vi "FIB profile.vi"(4 "Capella HV Data Output":T2 {"Column Vac (Torr)" format="%.2e"; "Gun Vac (Torr)" format="%.2e"; "Lens2 Actual (V)" format="%.1f"; "Lens1 Actual (V)" format="%.1f"; "Emission Actual (uA)" format="%.3f"; "Extrator Actual (V)" format="%.1f"; "Tip Lifetime (uAhr)" format="%.2f"; "Lens2 Target (V)" format="%.1f"; "Lens1 Target (V)" format="%.1f"; "SuppI (uA)" format="%.3f"; "Suppressor (V)" format="%.1f"; "Emission Target (uA)" format="%.3f"; "Extrator Target (V)" format="%.1f"; "Accelerator Actual (V)" format="%.1f"; "Accelerator Target (V)" format="%.1f"; "Filament (A)" format="%.2f"}, 5 "HV Data Output":T3 {"Tip Lifetime (hr)" format="%.2f"; "Lens2I (uA)" format="%.3f"; "Lens2 (V)" format="%.1f"; "Lens1I (uA)" format="%.3f"; "Lens1 (V)" format="%.1f"; "SuppI (uA)" format="%.3f"; "Suppressor (V)" format="%.1f"; "Emission (uA)" format="%.3f"; "Extrator (V)" format="%.1f"; "AccI (uA)" format="%.3f"; "Acclerator (V)" format="%.1f"; "Filament (A)" format="%.2f"}, 6 "Parameter Names":string[](array[string])=["Faraday Cup Current", "Specimen Current", "Beam Dump 1 Current", "Beam Dump 2 Current"], 7 "Active logging channels":string="Log/ai0:3", 8 "Scan Para":T5={"X resolution"=500, "Z resolution"=500, "X center"=0.0, "Z center"=0.0, "X size (V)"=10.0, "Z size (V)"=10.0, "Frame line rampdown ratio"=-0.1, "Scan rate (Hz)"=2000000, "Oversampling"=2} {"Frame line rampdown ratio" min=-1.0 max=1.0 step=0.05 format="%.2g"; "Scan rate (Hz)" max=4000000 format="%#.6p"}, 9 "Milling para":T1={"X resolution"=4096, "Z resolution"=125001, "X offset (um)"=0.0, "Z offset (um)"=0.0, "X center (um)"=0.0, "Z center (um)"=0.0, "X size (um)"=250.0, "Z size (um)"=250.0, "UL-Ang"=90.0, "UR-Ang"=90.0, "Line milling time (s)"=5.0, "Z-step (nm)"=2.0, "Lines auto pause"=1, "Auto pause"=FALSE, "Mill from Bottom"=FALSE, "FIB FOV (um)"=500.0, "Auto Profile"=FALSE, "Mill start from Last"=FALSE, "FIB PID on"=FALSE, "FIB PID reset"=TRUE, "FIB PID measured"=0, "FIB PID target"=0.0, "FIB PID target slope"=0.0, "FIB PID P"=0.001, "FIB PID I"=0.01, "FIB PID D"=0.0, "Emission (uA)"=1.36, "Suppressor (V)"=50.0, "Auto reheat"=FALSE} caption="Milling Parameters" {"Suppressor (V)" step=0.1 format="%.1g"; "Emission (uA)" step=0.1 format="%.2g"; "FIB PID measured" items=["Spec.", "B.D. 1", "B.D. 2", "Mill", "Spec. +"]; "FIB PID target slope" min=-1 max=1 step=0.1; "UR-Ang" format="%.2f"; "UL-Ang" format="%.2f"; "Z offset (um)" step=0.02 format="%.3g"; "X offset (um)" step=1 format="%.3g"; "FIB FOV (um)" format="%.3g"; "Line milling time (s)" format="%.1f"; "Z center (um)" format="%#.3g"; "X center (um)" format="%#.3g"}, 10 "Options":T6 {"Scan mode" items=["Raster", "Serpentine"]; "Det" items=["Detector A", "Detector B"]}, 11 "HW Config":T7={"FIB X coil"="FIB/ao0", "FIB Y coil"="FIB/ao1", "Beam blank"="FIB/port0/line0", "Ext Scan"="FIB/port0/line1", "Detector"="FIB/ai1", "Post #1up"="PXI1Slot2/ao0", "Post #1down"="PXI1Slot2/ao1", "Post #2up"="PXI1Slot2/ao2", "Post #2down"="PXI1Slot2/ao3"}) -> (0 "error out":errorcluster, 2 "Measurements":dbl[][](graph), 3 "Info & Status":T4={"Actual scan rate"=2000000.0, "X resolution with rampdown"=552, "Actual sample rate"=4000000.0, "Fetch backlog"=664878.0, "Total scan points"=276000, "Frame rate (/s)"=7} {"Fetch backlog" format="%#_6p"; "Actual sample rate" format="%#_6p"; "Actual scan rate" format="%#_4p"})   [LabVIEW 2018]
uses:
  <vilib>/DAQmx/write.llb/DAQmx Write (Digital Wfm 1Chan NSamp).vi
  <vilib>/DAQmx/write.llb/DAQmx Write (Analog 2D DBL NChan NSamp).vi
  <vilib>/DAQmx/read.llb/DAQmx Read (Analog 2D DBL NChan NSamp).vi
  <vilib>/DAQmx/create/channels.llb/DAQmx Create Channel (AI-Voltage-Basic).vi
  <vilib>/Waveform/DWDTOps.llb/DWDT Invert Digital.vi
  <vilib>/DAQmx/create/channels.llb/DAQmx Create Channel (AO-Voltage-Basic).vi
  <vilib>/DAQmx/create/channels.llb/DAQmx Create Channel (DO-Digital Output).vi
  <vilib>/Waveform/DWDTOps.llb/Digital Pattern Generator (Single Value).vi
  <vilib>/Waveform/DWDTOps.llb/DWDT Replace Subset.vi
  <vilib>/DAQmx/configure/timing.llb/DAQmx Timing (Sample Clock).vi
  <vilib>/DAQmx/create/channels.llb/DAQmx Create Channel (CO-Pulse Generation-Frequency).vi
  <vilib>/DAQmx/configure/trigger.llb/DAQmx Start Trigger (Digital Edge).vi
  <vilib>/Waveform/DWDTOps.llb/DWDT Uncompress Digital.vi
  <vilib>/DAQmx/miscellaneous.llb/DAQmx Fill In Error Info.vi
  <vilib>/Utility/file.llb/Write To Spreadsheet File (string).vi
  <resource>/objmgr/daqmx.rc
panel:
  out "Blanking":digitalwaveform(graph)
  in  "Api":refnum<k7>(container)
  in  "COM port":refnum<visa-resource-name>="COM1"
  out "Mill from Bottom":bool
  out "Y scan pattern":dbl[](array[numeric])
  out "AI SampleClk.MaxRate":dbl
  in  "Machine Type":u8(ring) items=["Feiss", "NVision", "Jeiss"]
  out "Ext scan":tag
  out "FIB Y coil":tag="PXI1Slot7/ao1"
  out "FIB X coil":tag="PXI1Slot7/ao0"
  in  "Beam blanked":bool
  out "Beam blank":tag="PXI1Slot7/port0/line0"
  out "Oversampling":u16=2
  out "Frame line rampdown ratio":dbl=0.1
  out "Y end":dbl=1.0
  out "X end":dbl=1.0
  out "Y start":dbl=-1.0
  out "X start":dbl=-1.0
  out "Y resolution":u32=500
  out "X resolution":u32=500
  out "Flip z":bool
  out "Flip x":bool
  out "Scan mode":u16
  in  "stop":bool=TRUE
  # "Direction"
  # "Start\nfrom"
  # "<"
  # "Flip"
  # "Scan coils"
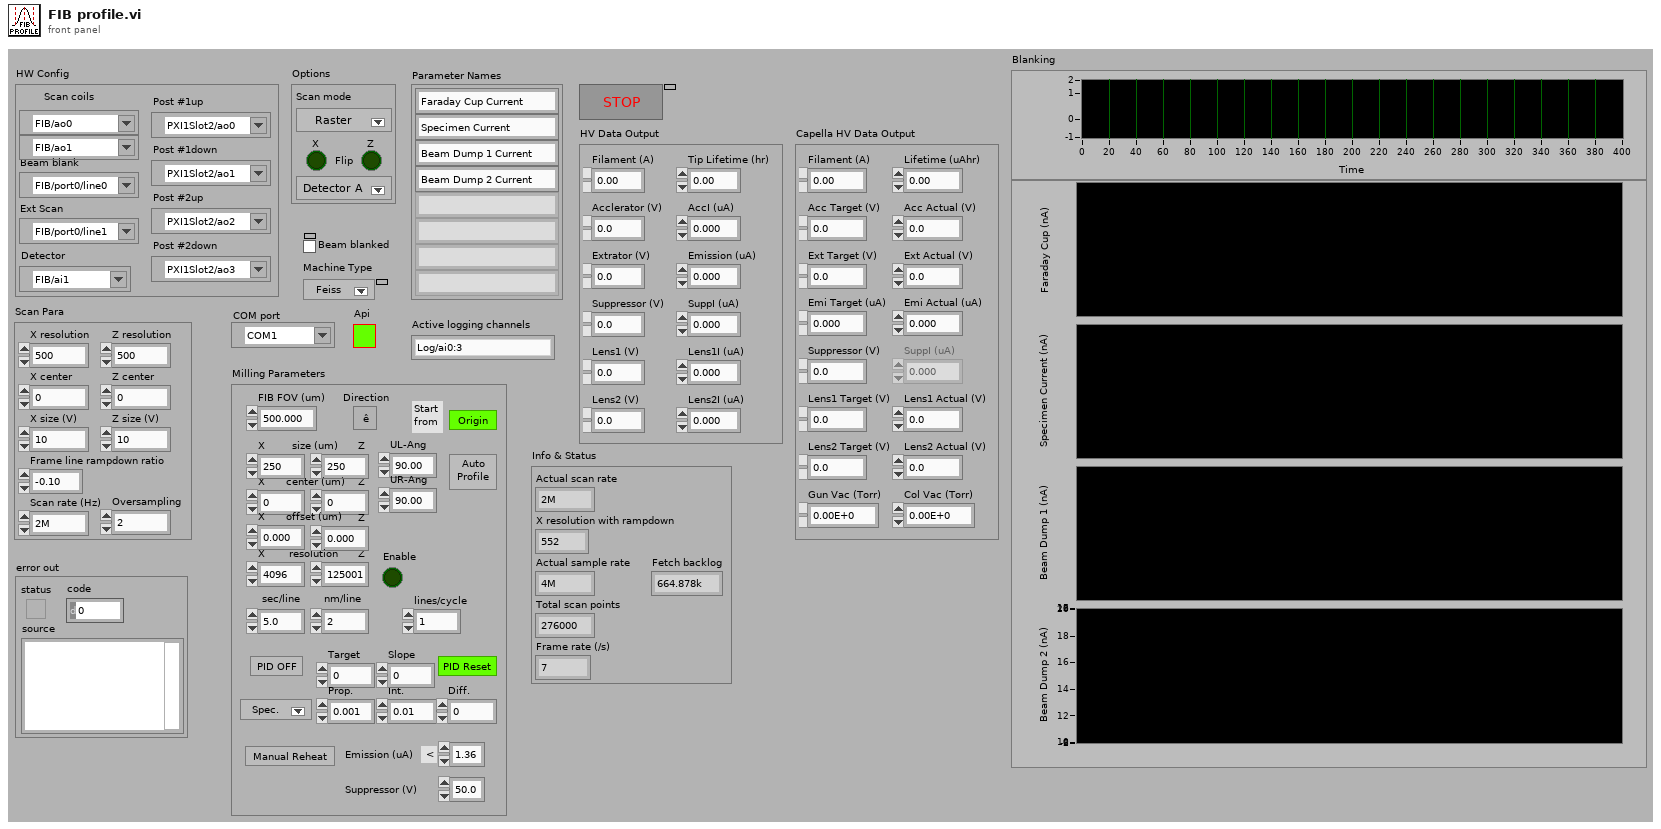
[diagram p1: front panel]
types:
  T1 = cluster{"X resolution":u32, "Z resolution":u32, "X offset (um)":sgl, "Z offset (um)":sgl, "X center (um)":sgl, "Z center (um)":sgl, "X size (um)":sgl, "Z size (um)":sgl, "UL-Ang":sgl, "UR-Ang":sgl, "Line milling time (s)":sgl, "Z-step (nm)":dbl, "Lines auto pause":u16, "Auto pause":bool, "Mill from Bottom":bool, "FIB FOV (um)":sgl, "Auto Profile":bool, "Mill start from Last":bool, "FIB PID on":bool, "FIB PID reset":bool, "FIB PID measured":u8, "FIB PID target":sgl, "FIB PID target slope":sgl, "FIB PID P":sgl, "FIB PID I":sgl, "FIB PID D":sgl, "Emission (uA)":dbl, "Suppressor (V)":sgl, "Auto reheat":bool}
  T2 = cluster{"Filament (A)":sgl, "Accelerator Target (V)":sgl, "Accelerator Actual (V)":sgl, "Extrator Target (V)":sgl, "Extrator Actual (V)":sgl, "Emission Target (uA)":sgl, "Emission Actual (uA)":sgl, "Suppressor (V)":sgl, "SuppI (uA)":sgl, "Lens1 Target (V)":sgl, "Lens1 Actual (V)":sgl, "Lens2 Target (V)":sgl, "Lens2 Actual (V)":sgl, "Gun Vac (Torr)":sgl, "Column Vac (Torr)":sgl, "Tip Lifetime (uAhr)":sgl}
  T3 = cluster{"Filament (A)":sgl, "Acclerator (V)":sgl, "AccI (uA)":sgl, "Extrator (V)":sgl, "Emission (uA)":sgl, "Suppressor (V)":sgl, "SuppI (uA)":sgl, "Lens1 (V)":sgl, "Lens1I (uA)":sgl, "Lens2 (V)":sgl, "Lens2I (uA)":sgl, "Tip Lifetime (hr)":sgl}
  T4 = cluster{"Actual scan rate":dbl, "X resolution with rampdown":i32, "Actual sample rate":dbl, "Fetch backlog":dbl, "Total scan points":i32, "Frame rate (/s)":u32}
  T5 = cluster{"X resolution":u32, "Z resolution":u32, "X center":dbl, "Z center":dbl, "X size (V)":dbl, "Z size (V)":dbl, "Frame line rampdown ratio":dbl, "Scan rate (Hz)":u32, "Oversampling":u16}
  T6 = cluster{"Scan mode":u16, "Flip x":bool, "Flip z":bool, "Det":u16}
  T7 = cluster{"FIB X coil":tag, "FIB Y coil":tag, "Beam blank":tag, "Ext Scan":tag, "Detector":tag, "Post #1up":tag, "Post #1down":tag, "Post #2up":tag, "Post #2down":tag}
  T8 = enum16{"SEM", "FIB", "Milling", "SEM + FIB", "Mill + SEM", "SEM Drift Correction", "FIB Drift Correction", "No Beam", "External", "External + SEM"}
  T9 = enum16{"SEM", "FIB", "Mill", "SEM + FIB", "Mill + SEM", "Drift SEM", "Drift FIB", "None", "Ext", "Ext + SEM"}
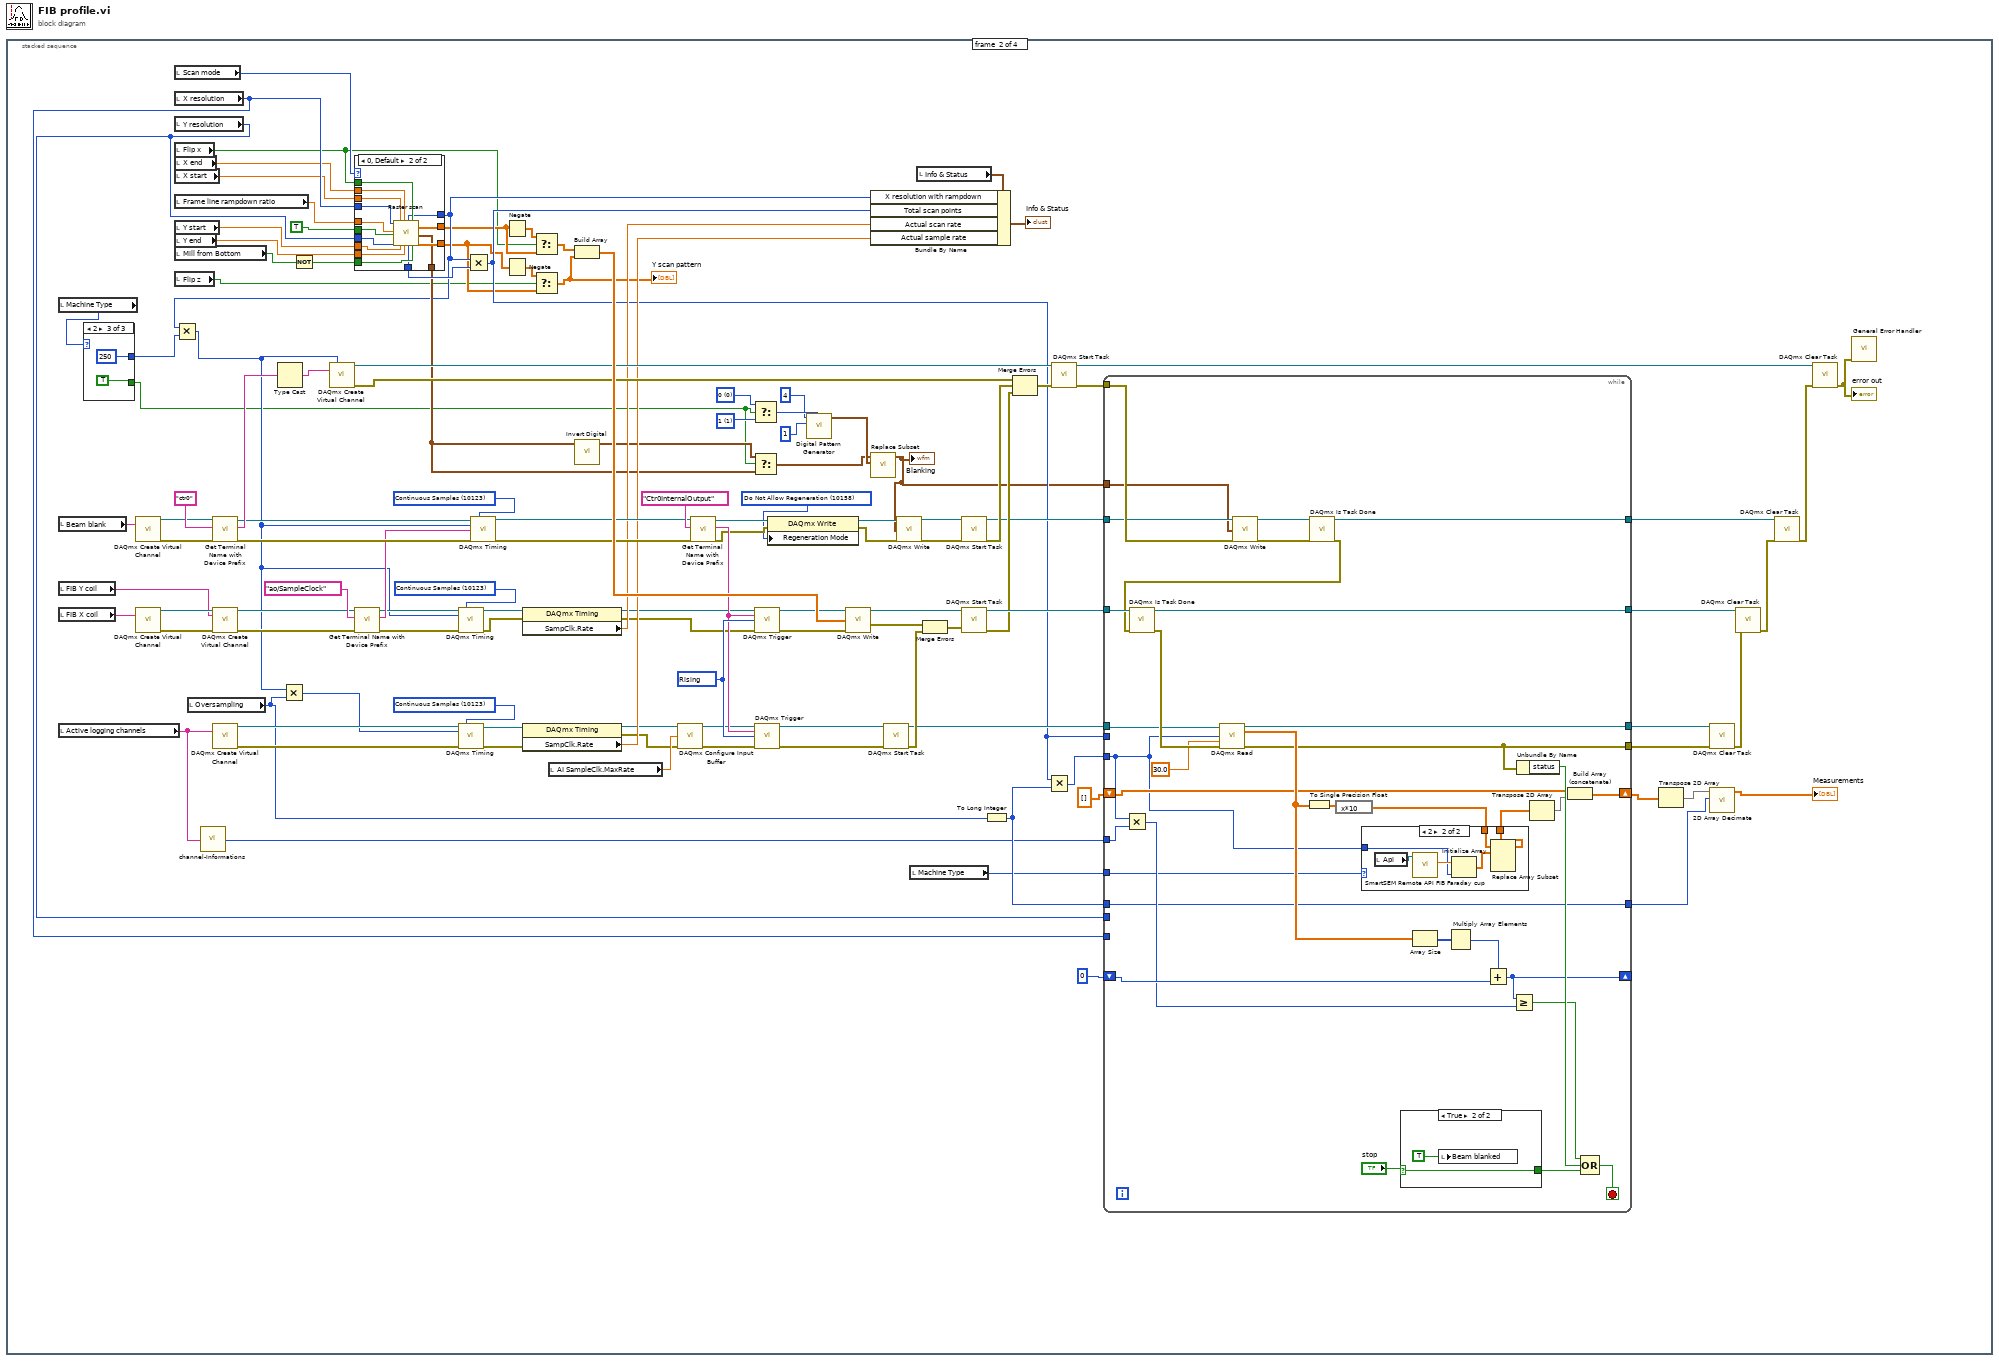
[diagram p0: block diagram]
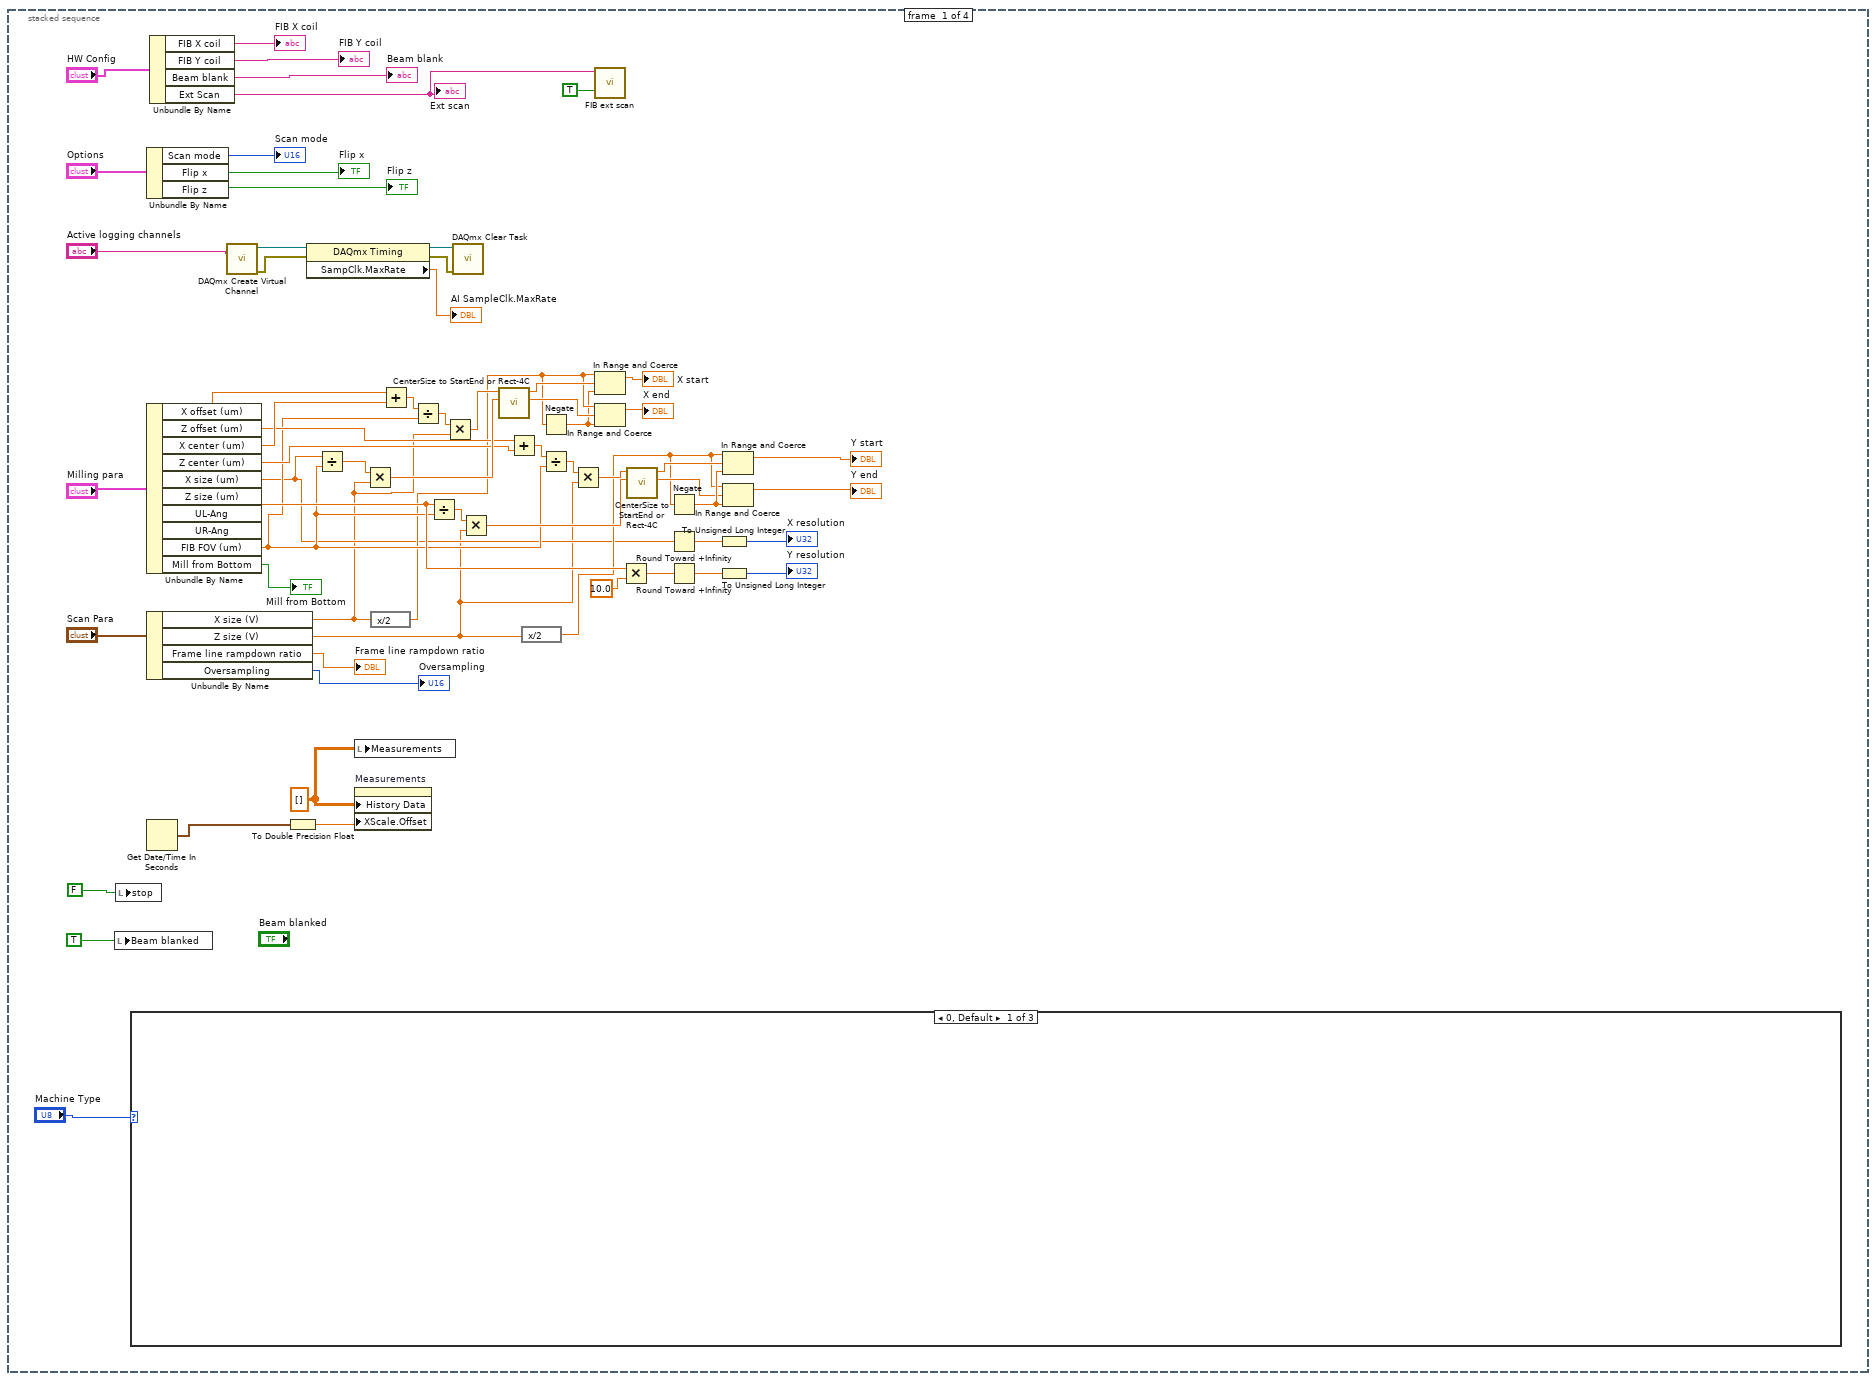
[diagram p2: hidden frame]
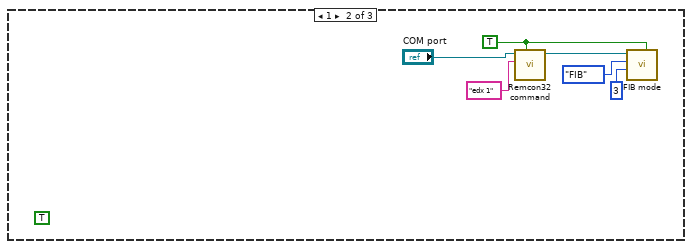
[diagram p3: hidden frame]
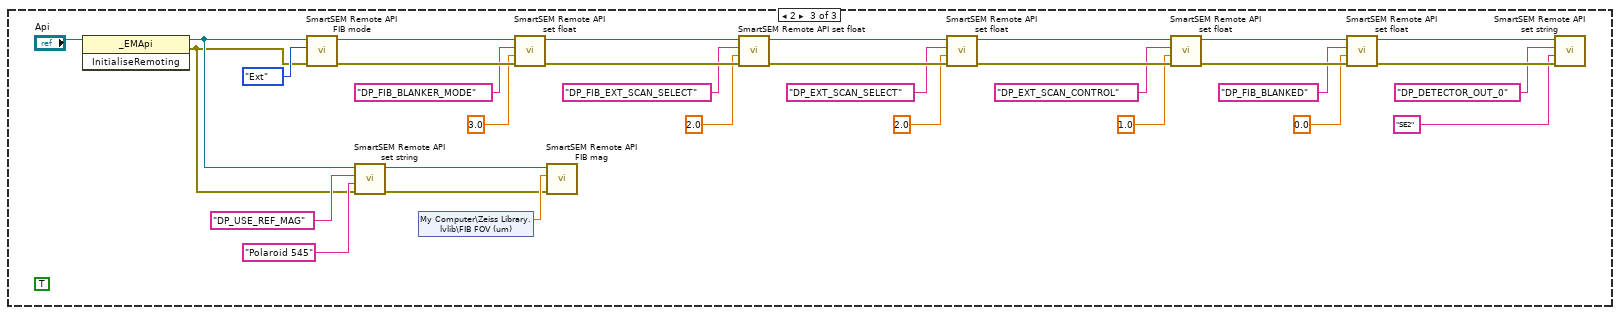
[diagram p4: hidden frame]
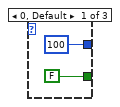
[diagram p5: hidden frame]
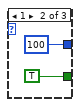
[diagram p6: hidden frame]
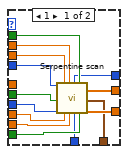
[diagram p7: hidden frame]
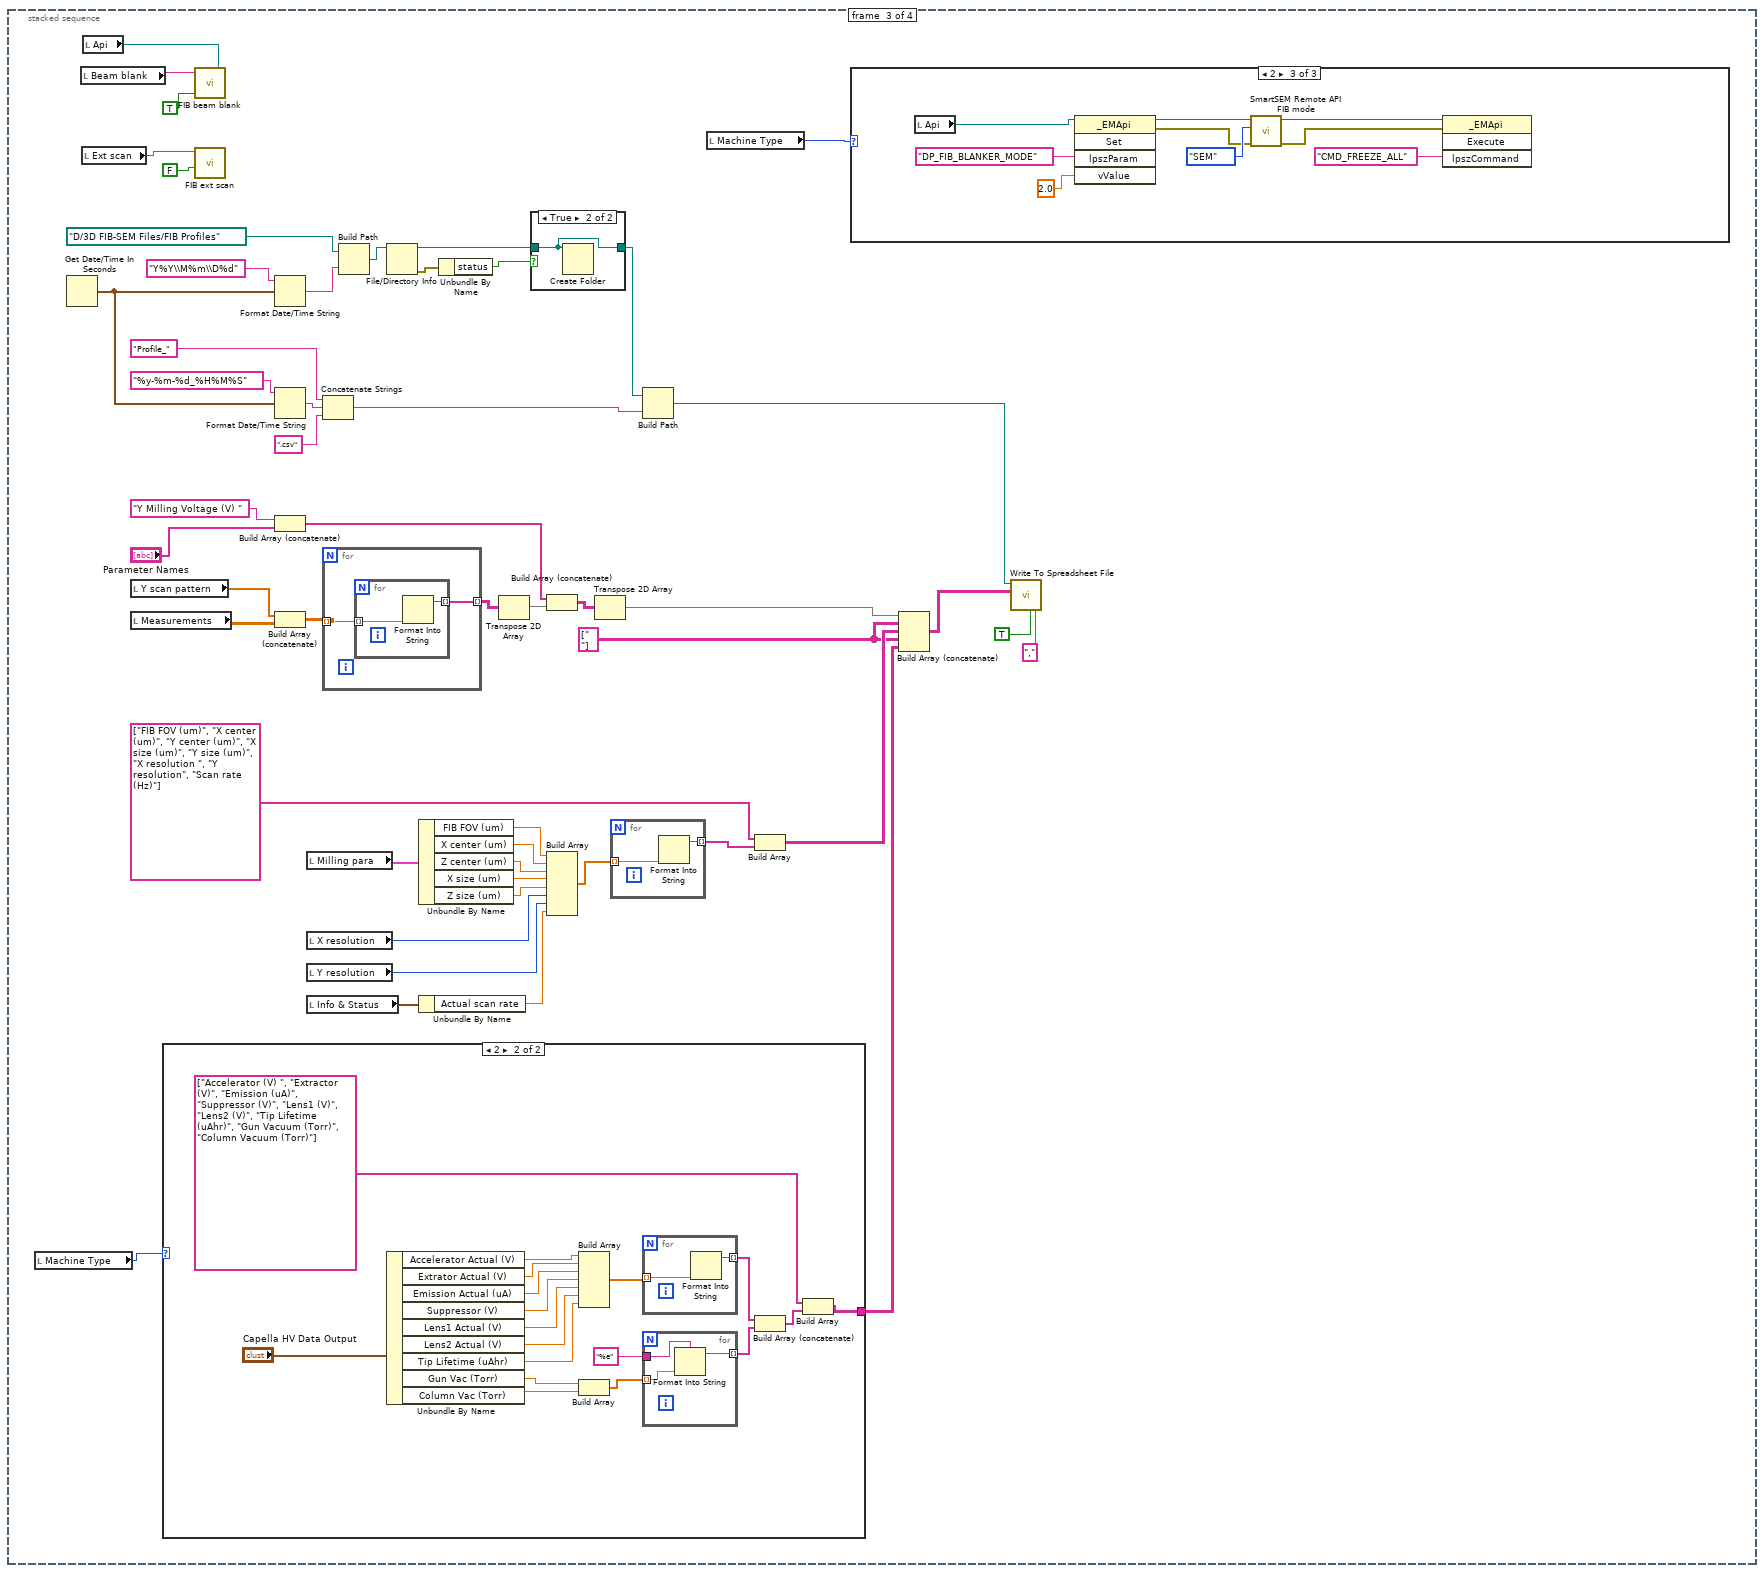
[diagram p10: hidden frame]
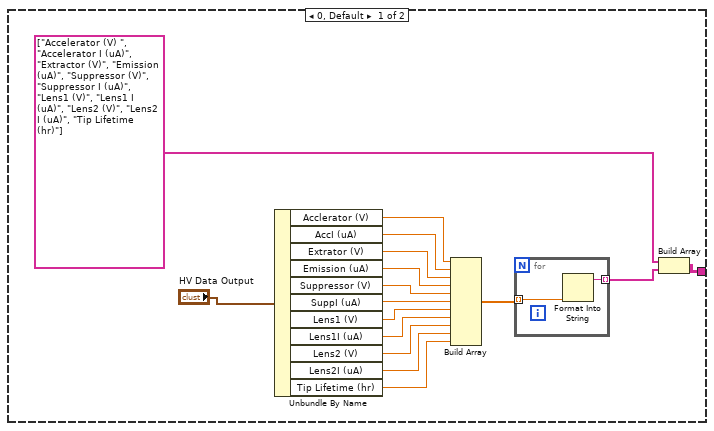
[diagram p11: hidden frame]
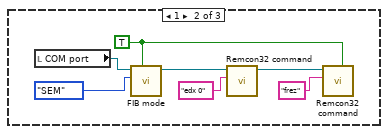
[diagram p13: hidden frame]
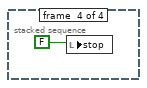
[diagram p15: hidden frame]
diagram:
  n1 = stacked-sequence {
    frame #0 {
      w7 = dbl[][] [] ("History Data")
      n2 = local write "Beam blanked"(TRUE ("Beam blanked")) -> ()
      n3 = local write "stop"(FALSE ("stop")) -> ()
      n4 = case shown="0, Default" "Machine Type" {
        frame 0, Default {
        }
        frame 1 {
          w68 = TRUE ("Close session")
          (unwired) TRUE ("Beam blanked")
          n5 = call "Remcon32 command.vi"("Initialization"=w68, "SEM command"="edx 1", "COM port in"="COM port") -> ("COM port out"=w67:refnum<visa-resource-name>)  [unwired: 5 in, 3 out]
          n6 = call "FIB mode.vi"("Close session"=w68, "Iterations"=u32 3, "FIB mode"=T8."FIB", "COM port in"=w67) -> ()  [unwired: 6 in, 2 out]
        }
        frame 2 {
          (unwired) TRUE ("Beam blanked")
          n7 = invoke class="_EMApi" method="InitialiseRemoting"(reference="Api") -> (reference out=w79:refnum<k7>, error out=w78:errorcluster)  [unwired: 2 in, 1 out]
          n8 = call "SmartSEM Remote API FIB mode.vi"("error in"=w78, "FIB mode"=T9."Ext", "Api"=w79) -> ("error out"=w98:errorcluster, "Api out"=w99:refnum<k7>)  [unwired: 7 in]
          n9 = call "SmartSEM Remote API set string.vi"("error in"=w78, "vValue"="Polaroid 545" ("lpszParam"), "lpszParam"="DP_USE_REF_MAG", "Api"=w79) -> ("error out"=w71:errorcluster, "Api out"=w73:refnum<k7>)  [unwired: 6 in]
          n10 = shared-variable "My Computer\\Zeiss Library.lvlib\\FIB FOV (um)"() -> (w72:sgl)  [unwired: 1 in, 1 out]
          n11 = call "SmartSEM Remote API set float.vi"("error in"=w98, "vValue"=sgl 3.0, "lpszParam"="DP_FIB_BLANKER_MODE", "Api"=w99) -> ("error out"=w94:errorcluster, "Api out"=w95:refnum<k7>)  [unwired: 6 in]
          n12 = call "SmartSEM Remote API FIB mag.vi"("error in"=w71, "FIB FOV (um)"=w72, "Api"=w73) -> ()  [unwired: 7 in, 2 out]
          n13 = call "SmartSEM Remote API set float.vi"("error in"=w94, "vValue"=sgl 2.0, "lpszParam"="DP_FIB_EXT_SCAN_SELECT" ("lpszCommand"), "Api"=w95) -> ("error out"=w90:errorcluster, "Api out"=w91:refnum<k7>)  [unwired: 6 in]
          n14 = call "SmartSEM Remote API set float.vi"("vValue"=sgl 2.0, "lpszParam"="DP_EXT_SCAN_SELECT" ("lpszCommand")) -> ()  [unwired: 8 in, 2 out]
          n15 = call "SmartSEM Remote API set float.vi"("error in"=w90, "vValue"=sgl 1.0, "lpszParam"="DP_EXT_SCAN_CONTROL" ("lpszCommand"), "Api"=w91) -> ("error out"=w86:errorcluster, "Api out"=w87:refnum<k7>)  [unwired: 6 in]
          n16 = call "SmartSEM Remote API set float.vi"("error in"=w86, "vValue"=sgl 0.0, "lpszParam"="DP_FIB_BLANKED", "Api"=w87) -> ("error out"=w82:errorcluster, "Api out"=w83:refnum<k7>)  [unwired: 6 in]
          n17 = call "SmartSEM Remote API set string.vi"("error in"=w82, "vValue"="SE2" ("Det A Type"), "lpszParam"="DP_DETECTOR_OUT_0", "Api"=w83) -> ()  [unwired: 6 in, 2 out]
        }
      }
      n18 = Unbundle By Name("Options") -> ("Scan mode"=→"Scan mode":u16, "Flip x"=→"Flip x":bool, "Flip z"=→"Flip z":bool)
      n19 = Unbundle By Name("Milling para") -> ("X offset (um)"=w52:sgl, "Z offset (um)"=w48:sgl, "X center (um)"=w51:sgl, "Z center (um)"=w47:sgl, "X size (um)"=w14:sgl, "Z size (um)"=w40:sgl, "FIB FOV (um)"=w28:sgl, "Mill from Bottom"=→"Mill from Bottom":bool)  [unwired: 2 out]
      n20 = Unbundle By Name("Scan Para") -> ("X size (V)"=w3:dbl, "Z size (V)"=w4:dbl, "Frame line rampdown ratio"=→"Frame line rampdown ratio":dbl, "Oversampling"=→"Oversampling":u16)
      n21 = Get Date/Time In Seconds() -> (seconds since 1Jan1904=w9:timestamp)
      n22 = Unbundle By Name("HW Config") -> ("FIB X coil"=→"FIB X coil":tag, "FIB Y coil"=→"FIB Y coil":tag, "Beam blank"=→"Beam blank":tag, "Ext Scan"=w56:tag)
      "Ext scan" <- w56
      n23 = call-poly <vilib>:"DAQmx Create Virtual Channel.vi"("physical channels"="Active logging channels") -> ("task out"=w37:refnum<k21>, "error out"=w35:errorcluster)  [unwired: 8 in, 5 out]
      n24 = To Double Precision Float(number=w9) -> (double precision float=w8:dbl)
      n25 = property class="DAQmx Timing"(reference=w37, error in=w35) -> (reference out=w38:refnum<k21>, error out=w36:errorcluster, "SampClk.MaxRate"=→"AI SampleClk.MaxRate":dbl)
      n26 = Divide(x=w14, y=w28) -> (x/y=w53:sgl)
      n27 = local write "Measurements"(w7) -> ()
      n28 = property on="Measurements" class="WFChart (strict)"("History Data"=w7, "XScale.Offset"=w8) -> ()  [unwired: 2 in, 2 out]
      n29 = Multiply(x=w53, y=w3) -> (x*y=w49:dbl)
      n30 = expression code="x/2"(w3) -> (w23:dbl)
      n31 = Add(x=w52, y=w51) -> (x+y=w29:sgl)
      n32 = Divide(x=w29, y=w28) -> (x/y=w30:sgl)
      n33 = Divide(x=w40, y=w28) -> (x/y=w46:sgl)
      n34 = Multiply(x=w30, y=w3) -> (x*y=w50:dbl)
      n35 = call <vilib>:"DAQmx Clear Task.vi"("task in"=w38, "error in"=w36) -> ()  [unwired: 14 out]
      n36 = Multiply(x=w46, y=w4) -> (x*y=w44:dbl)
      n37 = call "CenterSize to StartEnd or Rect-4C.vi"("Size"=w49, "Center"=w50) -> ("End"=w25:dbl, "Start"=w27:dbl)  [unwired: 3 in, 1 out]
      n38 = Add(x=w48, y=w47) -> (x+y=w32:sgl)
      n39 = expression code="x/2"(w4) -> (w16:dbl)
      n40 = Negate(x=w23) -> (-x=w22:dbl)
      n41 = Divide(x=w32, y=w28) -> (x/y=w31:sgl)
      n42 = Multiply(x=w31, y=w4) -> (x*y=w45:dbl)
      n43 = call "FIB ext scan.vi"("Ext on"=TRUE ("data"), "FIB Ext Scan"=w56) -> ()  [unwired: 9 in, 1 out]
      n44 = In Range and Coerce(upper limit=w23, x=w27, lower limit=w22) -> (coerced(x)=→"X start":dbl)  [unwired: 1 out]
      n45 = In Range and Coerce(upper limit=w23, x=w25, lower limit=w22) -> (coerced(x)=→"X end":dbl)  [unwired: 1 out]
      n46 = Multiply(x=w40, y=sgl 10.0) -> (x*y=w15:sgl)
      n47 = call "CenterSize to StartEnd or Rect-4C.vi"("Size"=w44, "Center"=w45) -> ("End"=w17:dbl, "Start"=w18:dbl)  [unwired: 3 in, 1 out]
      n48 = Negate(x=w16) -> (-x=w21:dbl)
      n49 = Round Toward +Infinity(x=w14) -> (ceil(x): smallest int >= x=w13:sgl)
      n50 = Round Toward +Infinity(x=w15) -> (ceil(x): smallest int >= x=w12:sgl)
      n51 = To Unsigned Long Integer(number=w13) -> (unsigned 32bit integer=→"X resolution":u32)
      n52 = To Unsigned Long Integer(number=w12) -> (unsigned 32bit integer=→"Y resolution":u32)
      n53 = In Range and Coerce(upper limit=w16, x=w18, lower limit=w21) -> (coerced(x)=→"Y start":dbl)  [unwired: 1 out]
      n54 = In Range and Coerce(upper limit=w16, x=w17, lower limit=w21) -> (coerced(x)=→"Y end":dbl)  [unwired: 1 out]
    }
    frame #1 {
      w110 = u8 1 items=["0", "1", "Z", "L", "H", "X", "T", "V"] ("value")
      w147 = u8 0 items=["0", "1", "Z", "L", "H", "X", "T", "V"] ("value")
      w156 = 10158 items=["Allow Regeneration"=10097, "Do Not Allow Regeneration"=10158] ("RegenMode")
      w180 = 10123 items=["Finite Samples"=10178, "Continuous Samples"=10123] ("sample mode")
      w168 = 10280 items=["Rising"=10280, "Falling"=10171] ("edge")
      w205 = 10123 items=["Finite Samples"=10178, "Continuous Samples"=10123, "Hardware Timed Single Point"=12522] ("sample mode")
      w209 = 10123 items=["Finite Samples"=10178, "Continuous Samples"=10123, "Hardware Timed Single Point"=12522] ("sample mode")
      n55 = local read "Machine Type"() -> (w104:u8)
      n56 = local read "Beam blank"() -> (w152:tag)
      n57 = local read "FIB Y coil"() -> (w210:tag)
      n58 = local read "FIB X coil"() -> (w211:tag)
      n59 = local read "Active logging channels"() -> (w139:string)
      n60 = case shown="2" w104 {
        tunnel: [u32 100 ("x") u32 100 ("x") u32 250 ("x")] -> w103
        tunnel: [FALSE ("Flip x") TRUE ("Flip x") TRUE ("Flip x")] -> w102
        frame 0, Default {
        }
        frame 1 {
        }
        frame 2 {
        }
      }
      n61 = call-poly <vilib>:"DAQmx Create Virtual Channel.vi"("lines"=w152) -> ("task out"=w187:refnum<k21>, "error out"=w189:errorcluster)  [unwired: 6 in, 7 out]
      n62 = call-poly <vilib>:"DAQmx Create Virtual Channel.vi"("physical channels"=w211) -> ("task out"=w213:refnum<k21>, "error out"=w212:errorcluster)  [unwired: 8 in, 5 out]
      n63 = local read "Scan mode"() -> (w225:u16)
      n64 = local read "X resolution"() -> (w224:u32)
      n65 = local read "Y resolution"() -> (w223:u32)
      n66 = local read "Flip x"() -> (w112:bool)
      n67 = local read "X end"() -> (w216:dbl)
      n68 = local read "X start"() -> (w217:dbl)
      n69 = local read "Frame line rampdown ratio"() -> (w222:dbl)
      n70 = local read "Y start"() -> (w215:dbl)
      n71 = local read "Y end"() -> (w214:dbl)
      n72 = local read "Mill from Bottom"() -> (w121:bool)
      n73 = local read "Flip z"() -> (w117:bool)
      n74 = local read "Oversampling"() -> (w161:u16)
      n75 = call "channel-Informations.vi"("Channel Name"=w139) -> ("No. of channels:"=w138:i32)  [unwired: 2 out]
      n76 = call "Get Terminal Name with Device Prefix.vi"("error in"=w189, "Local Terminal Name"="ctr0", "task/channels in"=w187) -> ("error out"=w190:errorcluster, "Terminal Name with Device Prefix"=w192:tag, "task out"=w188:refnum<k21>)  [unwired: 6 in]
      n77 = call-poly <vilib>:"DAQmx Create Virtual Channel.vi"("task in"=w213, "physical channels"=w210, "error in"=w212) -> ("task out"=w144:refnum<k21>, "error out"=w143:errorcluster)  [unwired: 6 in, 5 out]
      n78 = call-poly <vilib>:"DAQmx Create Virtual Channel.vi"("physical channels"=w139) -> ("task out"=w207:refnum<k21>, "error out"=w206:errorcluster)  [unwired: 8 in, 5 out]
      n79 = Type Cast(x=w192) -> (*(type *) &x=w193:string)  [unwired: 1 in]
      n80 = Not(x=w121) -> (.not. x?=w111:bool)
      n81 = case shown="0, Default" w225 {
        tunnel: w222 -> [_ w259]
        tunnel: w112 -> [w242 w262]
        tunnel: w223 -> [w245 w257]
        tunnel: w224 -> [w247 w260]
        tunnel: w111 -> [w239 w261]
        tunnel: [w238 w256] -> w128
        tunnel: [w237 w255] -> w219
        tunnel: TRUE ("Flip x") -> [w246 w258]
        tunnel: w217 -> [w244 w254]
        tunnel: w216 -> [w243 w253]
        tunnel: w215 -> [w241 w252]
        tunnel: w214 -> [w240 w251]
        tunnel: [w236 w250] -> w113
        tunnel: [w235 w249] -> w119
        tunnel: [w234 w248] -> w145
        frame 1 {
          n82 = call "Serpentine scan.vi"("X resolution"=w247, "Scan pattern?"=w246, "Y resolution"=w245, "X start"=w244, "Y start"=w241, "X end"=w243, "Y end"=w240, "Flip x"=w242, "Flip y"=w239) -> ("X resolution with rampdown"=w238:i32, "Y resolution"=w237:i32, "X scan pattern"=w236:dbl[], "Blanking pattern"=w234:digitalwaveform, "Y scan pattern"=w235:dbl[])  [unwired: 3 in, 3 out]
        }
        frame 0, Default {
          n83 = call "Raster scan.vi"("X resolution"=w260, "Frame line rampdown ratio"=w259, "Scan pattern?"=w258, "Y resolution"=w257, "X start"=w254, "Y start"=w252, "X end"=w253, "Y end"=w251, "Flip x"=w262, "Flip y"=w261) -> ("X resolution with rampdown"=w256:i32, "Y resolution"=w255:i32, "X scan pattern"=w250:dbl[], "Blanking pattern"=w248:digitalwaveform, "Y scan pattern"=w249:dbl[])  [unwired: 2 in, 3 out]
        }
      }
      n84 = Multiply(x=w128, y=w103) -> (x*y=w129:u32)
      n85 = Multiply(x=w129, y=w161) -> (x*y=w162:u32)
      n86 = call-poly <vilib>:"DAQmx Create Virtual Channel.vi"("frequency"=w129, "counter"=w193) -> ("task out"=w183:refnum<k21>, "error out"=w185:errorcluster)  [unwired: 7 in, 5 out]
      n87 = call "Get Terminal Name with Device Prefix.vi"("error in"=w143, "Local Terminal Name"="ao/SampleClock", "task/channels in"=w144) -> ("error out"=w163:errorcluster, "Terminal Name with Device Prefix"=w176:tag, "task out"=w164:refnum<k21>)  [unwired: 6 in]
      n88 = call-poly <vilib>:"DAQmx Timing.vi"("task/channels in"=w164, "sample mode"=w209, "rate"=w129, "error in"=w163) -> ("task out"=w166:refnum<k21>, "error out"=w165:errorcluster)  [unwired: 3 in, 7 out]
      n89 = call-poly <vilib>:"DAQmx Timing.vi"("task/channels in"=w207, "sample mode"=w205, "rate"=w162, "error in"=w206) -> ("task out"=w204:refnum<k21>, "error out"=w203:errorcluster)  [unwired: 3 in, 7 out]
      n90 = Multiply(x=w128, y=w219) -> (x*y=w127:i32)
      n91 = call-poly <vilib>:"DAQmx Timing.vi"("task/channels in"=w188, "sample mode"=w180, "rate"=w129, "source"=w176, "error in"=w190) -> ("task out"=w179:refnum<k21>, "error out"=w178:errorcluster)  [unwired: 2 in, 7 out]
      n92 = Negate(x=w113) -> (-x=w115:dbl[])
      n93 = Negate(x=w119) -> (-x=w120:dbl[])
      n94 = property class="DAQmx Timing"(reference=w166, error in=w165) -> (reference out=w149:refnum<k21>, error out=w148:errorcluster, "SampClk.Rate"=w151:dbl)
      n95 = property class="DAQmx Timing"(reference=w204, error in=w203) -> (reference out=w135:refnum<k21>, error out=w134:errorcluster, "SampClk.Rate"=w150:dbl)
      n96 = Select(t=w115, s=w112, f=w113) -> (s? t:f=w114:dbl[])
      n97 = Select(t=w120, s=w117, f=w119) -> (s? t:f=w118:dbl[])
      "Y scan pattern" <- w118
      n98 = local read "AI SampleClk.MaxRate"() -> (w137:dbl)
      n99 = Build Array(w114, w118) -> (w201:dbl[][])
      n100 = call-poly <vilib>:"Invert Digital.vi"("digital waveform"=w145) -> ("inverted waveform"=w146:digitalwaveform)  [unwired: 9 in, 1 out]
      n101 = call <vilib>:"DAQmx Configure Input Buffer.vi"("task/channels in"=w135, "buffer size (in samples per channel)"=w137, "error in"=w134) -> ("task out"=w136:refnum<k21>, "error out"=w133:errorcluster)  [unwired: 11 in]
      n102 = call "Get Terminal Name with Device Prefix.vi"("error in"=w178, "Local Terminal Name"="Ctr0InternalOutput" ("terminal"), "task/channels in"=w179) -> ("error out"=w158:errorcluster, "Terminal Name with Device Prefix"=w167:tag, "task out"=w160:refnum<k21>)  [unwired: 1 in, 5 out]
      n103 = Select(t=w147, s=w102, f=w110) -> (s? t:f=w109:u8)
      n104 = Select(t=w146, s=w102, f=w145) -> (s? t:f=w106:digitalwaveform)
      n105 = call-poly <vilib>:"DAQmx Trigger.vi"("task/channels in"=w149, "source"=w167, "edge"=w168, "error in"=w148) -> ("task out"=w169:refnum<k21>, "error out"=w170:errorcluster)  [unwired: 10 out]
      n106 = call-poly <vilib>:"DAQmx Trigger.vi"("task/channels in"=w136, "source"=w167, "edge"=w168, "error in"=w133) -> ("task out"=w140:refnum<k21>, "error out"=w202:errorcluster)  [unwired: 10 out]
      n107 = property class="DAQmx Write"(reference=w160, error in=w158, "Regeneration Mode"=w156) -> (reference out=w159:refnum<k21>, error out=w157:errorcluster)
      n108 = call-poly <vilib>:"Digital Pattern Generator.vi"("value"=w109, "number of signals"=u32 1, "number of samples"=u32 4) -> ("digital waveform"=w107:digitalwaveform)  [unwired: 2 in, 6 out]
      n109 = call-poly <vilib>:"DAQmx Write.vi"("task/channels in"=w169, "data"=w201, "error in"=w170) -> ("task out"=w200:refnum<k21>, "error out"=w198:errorcluster)  [unwired: 1 in, 10 out]
      n110 = call-poly <vilib>:"Replace Subset.vi"("new digital waveform"=w107, "digital waveform in"=w106) -> ("digital waveform out"=w105:digitalwaveform)  [unwired: 7 in, 2 out]
      "Blanking" <- w105
      n111 = call <vilib>:"DAQmx Start Task.vi"("task/channels in"=w140, "error in"=w202) -> ("task out"=w130:refnum<k21>, "error out"=w197:errorcluster)  [unwired: 12 out]
      n112 = call-poly <vilib>:"DAQmx Write.vi"("task/channels in"=w159, "data"=w105, "error in"=w157) -> ("task out"=w182:refnum<k21>, "error out"=w177:errorcluster)  [unwired: 2 in, 9 out]
      n113 = local read "Machine Type"() -> (w116:u8)
      n114 = local read "Info & Status"() -> (w221:T4)
      n115 = Bundle By Name(cluster=w221, "X resolution with rampdown"=w128, "Total scan points"=w127, "Actual scan rate"=w151, "Actual sample rate"=w150) -> (→"Info & Status":T4)
      n116 = Merge Errors(w198, w197) -> (w199:errorcluster)
      n117 = call <vilib>:"DAQmx Start Task.vi"("task/channels in"=w182, "error in"=w177) -> ("task out"=w173:refnum<k21>, "error out"=w184:errorcluster)  [unwired: 12 out]
      n118 = call <vilib>:"DAQmx Start Task.vi"("task/channels in"=w200, "error in"=w199) -> ("task out"=w196:refnum<k21>, "error out"=w175:errorcluster)  [unwired: 12 out]
      n119 = To Long Integer(number=w161) -> (32bit integer=w227:i32)
      n120 = Merge Errors(w185, w184, w175) -> (w186:errorcluster)
      n121 = Multiply(x=w127, y=w227) -> (x*y=w226:i32)
      n122 = call <vilib>:"DAQmx Start Task.vi"("task/channels in"=w183, "error in"=w186) -> ("task out"=w172:refnum<k21>, "error out"=w174:errorcluster)  [unwired: 12 out]
      n123 = while {
        tunnel: w227 -> [w268]
        tunnel: w223 -> [_]
        tunnel: w224 -> [_]
        tunnel: w226 -> [w265]
        tunnel: w130 -> [w280]
        tunnel: w196 -> [w294]
        tunnel: [w273] -> w131
        tunnel: [w274] -> w132
        tunnel: [w293] -> w195
        tunnel: w174 -> [w288]
        tunnel: w173 -> [w287]
        tunnel: [w290] -> w171
        tunnel: w105 -> [w263]
        shift-right: [w284] -> _
        shift-left: 0 -> [w285]
        tunnel: w138 -> [w279]
        tunnel: w127 -> [_]
        shift-right: [w271] -> w126
        shift-left: sgl[][] [] -> [w269]
        tunnel: [w268] -> w122
        tunnel: w116 -> [w264]
        stop <- w297 stop-if-true
        n124 = Multiply(x=w265, y=w279) -> (x*y=w275:i32)
        n125 = call-poly <vilib>:"DAQmx Write.vi"("task/channels in"=w287, "data"=w263, "error in"=w288) -> ("task out"=w286:refnum<k21>, "error out"=w289:errorcluster)  [unwired: 2 in, 9 out]
        n126 = call <vilib>:"DAQmx Is Task Done.vi"("task/channels in"=w286, "error in"=w289) -> ("task out"=w290:refnum<k21>, "error out"=w291:errorcluster)  [unwired: 2 in, 10 out]
        n127 = call <vilib>:"DAQmx Is Task Done.vi"("task/channels in"=w294, "error in"=w291) -> ("task out"=w293:refnum<k21>, "error out"=w281:errorcluster)  [unwired: 2 in, 10 out]
        n128 = call-poly <vilib>:"DAQmx Read.vi"("task/channels in"=w280, "number of samples per channel"=w265, "timeout"=30.0, "error in"=w281) -> ("task out"=w274:refnum<k21>, "data"=w278:dbl[][], "error out"=w273:errorcluster)  [unwired: 9 out]
        n129 = To Single Precision Float(number=w278) -> (single precision float=w282:sgl[][])
        n130 = expression code="x*10"(w282) -> (w267:sgl[][])
        n131 = case shown="2" w264 {
          tunnel: w267 -> [w298 w301]
          tunnel: w265 -> [_ w300]
          tunnel: [w298 w299] -> w266
          frame 0, Default {
          }
          frame 2 {
            n132 = local read "Api"() -> (w302:refnum<k7>)
            n133 = call "SmartSEM Remote API FIB Faraday cup.vi"("Api"=w302) -> ("FIB Faraday Cup (nA)"=w303:sgl)  [unwired: 8 in, 2 out]
            n134 = Initialize Array(w303, w300) -> (w304:sgl[])
            n135 = Replace Array Subset(array=w301, new element=w304) -> (w299:sgl[][])  [unwired: 2 in]
          }
        }
        n136 = case shown="True" "stop" {
          selector: "stop" -> [w305 w307]
          tunnel: [w305 w307] -> w295
          frame False {
          }
          frame True {
            n137 = local write "Beam blanked"(TRUE ("Beam blanked")) -> ()
          }
        }
        n138 = Array Size(array=w278) -> (size(s)=w277:i32[])
        n139 = Multiply Array Elements(1:w277) -> (0:w276:i32)
        n140 = Add(x=w276, y=w285) -> (x+y=w284:i32)
        n141 = Greater Or Equal?(x=w284, y=w275) -> (x >= y?=w283:bool)
        n142 = Unbundle By Name(w273) -> ("status"=w292:bool)
        n143 = Transpose 2D Array(2D array=w266) -> (transposed array=w270:sgl[][])
        n144 = Build Array (concatenate)(w269, w270) -> (w271:sgl[][])
        n145 = Compound Arithmetic op=OR(w283, w292, w295) -> (w297:bool)
      }
      n146 = Transpose 2D Array(2D array=w126) -> (transposed array=w124:sgl[][])
      n147 = call <vilib>:"DAQmx Clear Task.vi"("task in"=w132, "error in"=w131) -> ("error out"=w194:errorcluster)  [unwired: 13 out]
      n148 = call "2D Array Decimate.vi"("x decimating factor"=w122, "Input 2D Array"=w124) -> ("output array"=→"Measurements":dbl[][])  [unwired: 7 in, 2 out]
      n149 = call <vilib>:"DAQmx Clear Task.vi"("task in"=w195, "error in"=w194) -> ("error out"=w154:errorcluster)  [unwired: 13 out]
      n150 = call <vilib>:"DAQmx Clear Task.vi"("task in"=w171, "error in"=w154) -> ("error out"=w153:errorcluster)  [unwired: 13 out]
      n151 = call <vilib>:"DAQmx Clear Task.vi"("task in"=w172, "error in"=w153) -> ("error out"=w141:errorcluster)  [unwired: 13 out]
      "error out" <- w141
      n152 = call <vilib>:"General Error Handler.vi"("error in (no error)"=w141) -> ()  [unwired: 10 in, 5 out]
    }
    frame #2 {
      w312 = string[][] [[" "]] ("array")
      n153 = local read "Machine Type"() -> (w309:u8)
      n154 = Get Date/Time In Seconds() -> (seconds since 1Jan1904=w347:timestamp)
      n155 = local read "Beam blank"() -> (w357:tag)
      n156 = local read "Ext scan"() -> (w356:tag)
      n157 = local read "Api"() -> (w308:refnum<k7>)
      n158 = local read "Y scan pattern"() -> (w339:dbl[])
      n159 = local read "Measurements"() -> (w340:dbl[][])
      n160 = case shown="2" w309 {
        tunnel: [w359 w380] -> w311
        frame 0, Default {
          n161 = Unbundle By Name("HV Data Output") -> ("Acclerator (V)"=w373:sgl, "AccI (uA)"=w372:sgl, "Extrator (V)"=w371:sgl, "Emission (uA)"=w370:sgl, "Suppressor (V)"=w369:sgl, "SuppI (uA)"=w368:sgl, "Lens1 (V)"=w367:sgl, "Lens1I (uA)"=w366:sgl, "Lens2 (V)"=w365:sgl, "Lens2I (uA)"=w364:sgl, "Tip Lifetime (hr)"=w363:sgl)
          n162 = Build Array(w373, w372, w371, w370, w369, w368, w367, w366, w365, w364, w363) -> (w362:sgl[])
          n163 = for {
            tunnel: w362 -> [w376] mode=indexing
            tunnel: [w375] -> w361 mode=indexing
            n164 = Format Into String(w376) -> (resulting string=w375:string)  [unwired: 3 in, 1 out]
          }
          n165 = Build Array(string[] ["Accelerator (V) ", "Accelerator I (uA)", "Extractor (V)", "Emission (uA)", "Suppressor (V)", "Suppressor I (uA)", "Lens1 (V)", "Lens1 I (uA)", "Lens2 (V)", "Lens2 I (uA)", "Tip Lifetime (hr)"] ("Parameter Names"), w361) -> (w359:string[][])
        }
        frame 2 {
          n166 = Unbundle By Name("Capella HV Data Output") -> ("Accelerator Actual (V)"=w394:sgl, "Extrator Actual (V)"=w393:sgl, "Emission Actual (uA)"=w392:sgl, "Suppressor (V)"=w391:sgl, "Lens1 Actual (V)"=w390:sgl, "Lens2 Actual (V)"=w389:sgl, "Tip Lifetime (uAhr)"=w385:sgl, "Gun Vac (Torr)"=w382:sgl, "Column Vac (Torr)"=w381:sgl)
          n167 = Build Array(w394, w393, w392, w391, w390, w389, w385) -> (w388:sgl[])
          n168 = Build Array(w382, w381) -> (w384:sgl[])
          n169 = for {
            tunnel: w388 -> [w399] mode=indexing
            tunnel: [w398] -> w378 mode=indexing
            n170 = Format Into String(w399) -> (resulting string=w398:string)  [unwired: 3 in, 1 out]
          }
          n171 = for {
            tunnel: w384 -> [w397] mode=indexing
            tunnel: [w396] -> w377 mode=indexing
            tunnel: "%e" ("format string") -> [w395]
            n172 = Format Into String(format string=w395, w397) -> (resulting string=w396:string)  [unwired: 2 in, 1 out]
          }
          n173 = Build Array (concatenate)(w378, w377) -> (w379:string[])
          n174 = Build Array(string[] ["Accelerator (V) ", "Extractor (V)", "Emission (uA)", "Suppressor (V)", "Lens1 (V)", "Lens2 (V)", "Tip Lifetime (uAhr)", "Gun Vacuum (Torr)", "Column Vacuum (Torr)"] ("Parameter Names"), w379) -> (w380:string[][])
        }
      }
      n175 = call "FIB beam blank.vi"("Api"=w308, "Beam blanked"=TRUE, "lines"=w357) -> ()  [unwired: 2 in, 1 out]
      n176 = call "FIB ext scan.vi"("Ext on"=FALSE ("data"), "FIB Ext Scan"=w356) -> ()  [unwired: 9 in, 1 out]
      n177 = Format Date/Time String(time format string (%c)="Y%Y\\M%m\\D%d", seconds (now)=w347) -> (date/time string=w354:string)  [unwired: 1 out]
      n178 = Format Date/Time String(time format string (%c)="%y-%m-%d_%H%M%S", seconds (now)=w347) -> (date/time string=w346:string)  [unwired: 1 out]
      n179 = Build Array (concatenate)("Y Milling Voltage (V) " ("string"), "Parameter Names") -> (w331:string[])
      n180 = Build Array (concatenate)(w339, w340) -> (w338:dbl[][])
      n181 = local read "Milling para"() -> (w326:T1)
      n182 = local read "X resolution"() -> (w315:u32)
      n183 = local read "Y resolution"() -> (w314:u32)
      n184 = local read "Info & Status"() -> (w316:T4)
      n185 = Concatenate Strings("Profile_" ("string"), w346, ".csv" ("string")) -> (w344:string)
      n186 = for {
        tunnel: w338 -> [w419] mode=indexing
        tunnel: [w418] -> w333 mode=indexing
        n187 = for {
          tunnel: w419 -> [w421] mode=indexing
          tunnel: [w420] -> w418 mode=indexing
          n188 = Format Into String(w421) -> (resulting string=w420:string)  [unwired: 3 in, 1 out]
        }
      }
      n189 = Build Path(base path=path "D:/3D FIB-SEM Files/FIB Profiles" ("path"), name or relative path=w354) -> (appended path=w343:path)
      n190 = File/Directory Info(path=w343) -> (path out=w350:path, error out=w352:errorcluster)  [unwired: 1 in, 5 out]
      n191 = Unbundle By Name(w326) -> ("FIB FOV (um)"=w325:sgl, "X center (um)"=w324:sgl, "Z center (um)"=w323:sgl, "X size (um)"=w322:sgl, "Z size (um)"=w321:sgl)
      n192 = Unbundle By Name(w316) -> ("Actual scan rate"=w313:dbl)
      n193 = Unbundle By Name(w352) -> ("status"=w351:bool)
      n194 = Transpose 2D Array(2D array=w333) -> (transposed array=w332:string[][])
      n195 = case shown="True" w351 {
        tunnel: w350 -> [w422 w423]
        tunnel: [w422 w423] -> w342
        frame False {
        }
        frame True {
          n196 = Create Folder(path (use dialog)=w423) -> ()  [unwired: 1 in, 4 out]
        }
      }
      n197 = Build Array (concatenate)(w331, w332) -> (w328:string[][])
      n198 = Build Array(w325, w324, w323, w322, w321, w315, w314, w313) -> (w320:dbl[])
      n199 = Transpose 2D Array(2D array=w328) -> (transposed array=w329:string[][])
      n200 = for {
        tunnel: w320 -> [w417] mode=indexing
        tunnel: [w416] -> w318 mode=indexing
        n201 = Format Into String(w417) -> (resulting string=w416:string)  [unwired: 3 in, 1 out]
      }
      n202 = Build Path(base path=w342, name or relative path=w344) -> (appended path=w336:path)
      n203 = local read "Machine Type"() -> (w310:u8)
      n204 = Build Array(string[] ["FIB FOV (um)", "X center (um)", "Y center (um)", "X size (um)", "Y size (um)", "X resolution ", "Y resolution", "Scan rate (Hz)"] ("Parameter Names"), w318) -> (w317:string[][])
      n205 = case shown="2" w310 {
        frame 0, Default {
        }
        frame 1 {
          w406 = TRUE ("Initialization")
          n206 = local read "COM port"() -> (w400:refnum<visa-resource-name>)
          n207 = call "FIB mode.vi"("Initialization"=w406, "FIB mode"=T8."SEM", "COM port in"=w400) -> ("COM port out"=w401:refnum<visa-resource-name>)  [unwired: 7 in, 1 out]
          n208 = call "Remcon32 command.vi"("SEM command"="edx 0", "COM port in"=w401) -> ("COM port out"=w402:refnum<visa-resource-name>)  [unwired: 6 in, 3 out]
          n209 = call "Remcon32 command.vi"("Close session"=w406, "SEM command"="frez", "COM port in"=w402) -> ()  [unwired: 5 in, 4 out]
        }
        frame 2 {
          n210 = local read "Api"() -> (w412:refnum<k7>)
          n211 = invoke class="_EMApi" method="Set"(reference=w412, "lpszParam"="DP_FIB_BLANKER_MODE" ("lpszCommand"), "vValue"=sgl 2.0) -> (reference out=w409:refnum<k7>, error out=w410:errorcluster)  [unwired: 2 in, 3 out]
          n212 = call "SmartSEM Remote API FIB mode.vi"("error in"=w410, "FIB mode"=T9."SEM", "Api"=w409) -> ("error out"=w407:errorcluster, "Api out"=w408:refnum<k7>)  [unwired: 7 in]
          n213 = invoke class="_EMApi" method="Execute"(reference=w408, error in=w407, "lpszCommand"="CMD_FREEZE_ALL") -> ()  [unwired: 1 in, 4 out]
        }
      }
      n214 = Build Array (concatenate)(w329, w312, w317, w312, w311) -> (w330:string[][])
      n215 = call-poly <vilib>:"Write To Spreadsheet File.vi"("delimiter (\\t)"="," ("delimiter (\\t)"), "transpose? (no:F)"=TRUE, "2D data"=w330, "file path (dialog if empty)"=w336) -> ()  [unwired: 4 in, 1 out]
    }
    frame #3 {
      n216 = local write "stop"(FALSE ("stop")) -> ()
    }
  }
